vi "Add Header.vi"(8 "error in (no error)":errorcluster, 9 "value":string, 10 "header":string, 11 "httpHeaders in":refnum<class "httpHeaders.lvclass">) -> (0 "error out":errorcluster, 3 "httpHeaders out":refnum<class "httpHeaders.lvclass">)   [LabVIEW 2020, in "httpClient.lvlib" / "httpHeaders.lvclass"]
uses:
  httpHeaders.lvclass
  httpHeaders.lvclass/httpHeaders.ctl
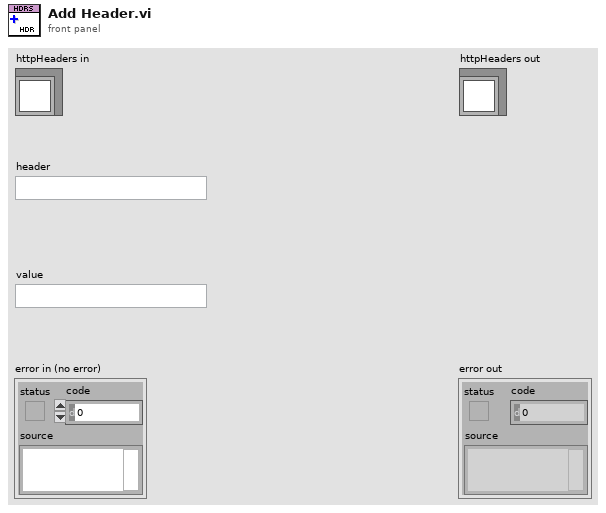
[diagram p1: front panel]
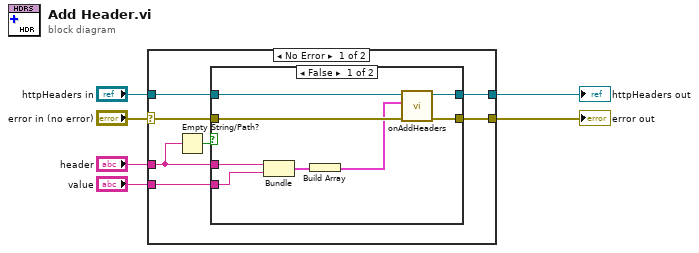
[diagram p0: block diagram]
diagram:
  n1 = case shown="No Error" "error in (no error)" {
    selector: "error in (no error)" -> [w13 w25]
    tunnel: [w12 w25] -> w5
    tunnel: [w11 w24] -> w3
    tunnel: "httpHeaders in" -> [w10 w24]
    tunnel: "header" -> [w8 _]
    tunnel: "value" -> [w9 _]
    frame No Error {
      n2 = Empty String/Path?(string/path=w8) -> (empty?=w7:bool)
      n3 = case shown="False" w7 {
        tunnel: w13 -> [w21 w22]
        tunnel: [w20 w22] -> w12
        tunnel: [w19 w23] -> w11
        tunnel: w10 -> [w18 w23]
        tunnel: w9 -> [w17 _]
        tunnel: w8 -> [w14 _]
        frame False {
          n4 = Bundle("header"=w14, "value"=w17) -> (w16:cluster{"header":string, "value":string})  [unwired: 1 in]
          n5 = Build Array(w16) -> (w15:cluster{"header":string, "value":string}[])
          n6 = call-dynamic "onAddHeaders.vi"("error in (no error)"=w21, "headers"=w15, "httpHeaders in"=w18) -> ("error out"=w20:errorcluster, "httpHeaders out"=w19:refnum<class "httpHeaders.lvclass">)  [unwired: 7 in]
        }
        frame True {
        }
      }
    }
    frame Error {
    }
  }
  "error out" <- w5
  "httpHeaders out" <- w3
